vi "Utility Parse Response.vi"(10 "error in (no error)":errorcluster, 11 "Response String":string) -> (2 "error out":errorcluster, 3 "Response Cluster":T1 {"Command ID" format="%x"})   [LabVIEW 2020, in "Omega Platinum Series.lvlib"]
doc: "Parses the controller response into a cluster with the unit address (-1 if none given), command class (G, P, R, or W), command ID (hex number), and parameter list (string)."
uses:
  Omega Platinum Series.lvlib
  Type Defs/Response.ctl
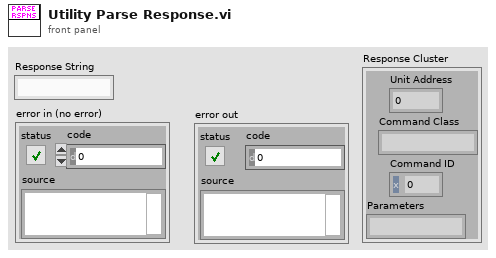
[diagram p1: front panel]
types:
  T1 = typedef "Omega Platinum Series.lvlib/Response.ctl" = cluster{"Unit Address":i32, "Command Class":string, "Command ID":u32, "Parameters":string}
  T2 = cluster{"default value 1":u32, string, "default value 1":u32, "trimmed string":string}
  T3 = cluster{"default value 1":i32, string, "default value 1":u32, "trimmed string":string}
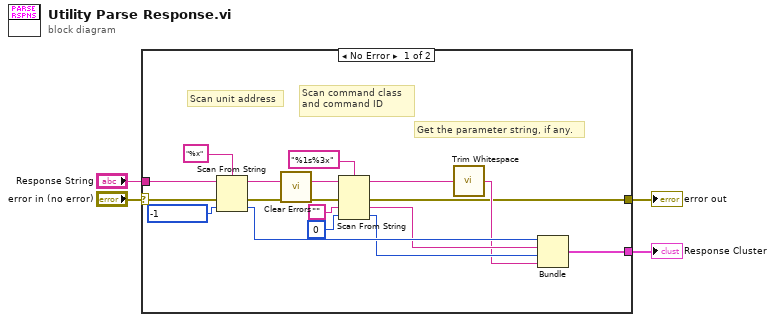
[diagram p0: block diagram]
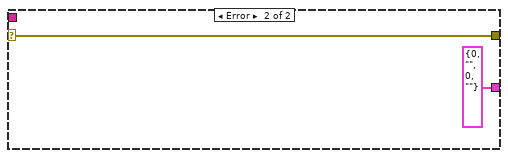
[diagram p2: hidden frame]
diagram:
  n1 = case shown="No Error" "error in (no error)" {
    selector: "error in (no error)" -> [w8 w23]
    tunnel: "Response String" -> [w21 _]
    tunnel: [w19 T2 {"default value 1"=0, "", "default value 1"=0, "trimmed string"=""}] -> w3
    tunnel: [w5 w23] -> w1
    frame No Error {
      # "Get the parameter string, if any."
      # "Scan command class\nand command ID"
      # "Scan unit address"
      n2 = Scan From String(format string="%x", input string=w21, error in=w8, default 1=-1 ("default value 1")) -> (remaining string=w18:string, error out=w7:errorcluster, output 1=w12:i32)  [unwired: 1 in, 1 out]
      n3 = call <vilib>:"Clear Errors.vi"("error in (no error)"=w7) -> ("error out"=w6:errorcluster)  [unwired: 5 in, 1 out]
      n4 = Scan From String(format string="%1s%3x", input string=w18, error in=w6, default 1="", default 2=u32 0 ("default value 1")) -> (remaining string=w14:string, error out=w5:errorcluster, output 1=w11:string, output 2=w10:u32)  [unwired: 1 in, 1 out]
      n5 = call <vilib>:"Trim Whitespace.vi"("string"=w14) -> ("trimmed string"=w9:string)  [unwired: 1 in]
      n6 = Bundle("default value 1"=w12, w11, "default value 1"=w10, "trimmed string"=w9) -> (w19:T3)  [unwired: 1 in]
    }
    frame Error {
    }
  }
  "error out" <- w1
  "Response Cluster" <- w3
